vi "rainbow.vi"() -> ()   [LabVIEW 2020]
uses:
  <vilib>/Rock Robotics/SystemInterfaces/DIO/FPGA_DIOPWMChannel.ctl
  Users/Adam/Downloads/bling-main/bling-main/BlingLibrary/ArduinoSerialBling.lvlib
panel:
  out "LED Strip":u32[](array[colorbox])
  out "String Length":u16=144
  in  "milliseconds to wait":u32
  in  "PWM Channel":T1=enum."PWM 9"
  in  "stop":bool
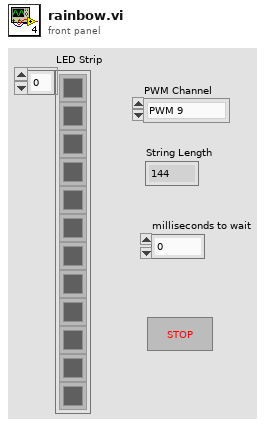
[diagram p1: front panel]
types:
  T1 = typedef "FPGA_DIOPWMChannel.ctl" = enum8{"PWM 0", "PWM 1", "PWM 2", "PWM 3", "PWM 4", "PWM 5", "PWM 6", "PWM 7", "PWM 8", "PWM 9", "PWM MXP 0", "PWM MXP 1", "PWM MXP 2", "PWM MXP 3", "PWM MXP 4", "PWM MXP 5", "PWM MXP 6", "PWM MXP 7", "PWM MXP 8", "PWM MXP 9", "Invalid"}
  T2 = typedef "WPI_PWMDeviceRef.ctl" = cluster{"DeviceStatus":errorcluster, "PWM Channel":T1}
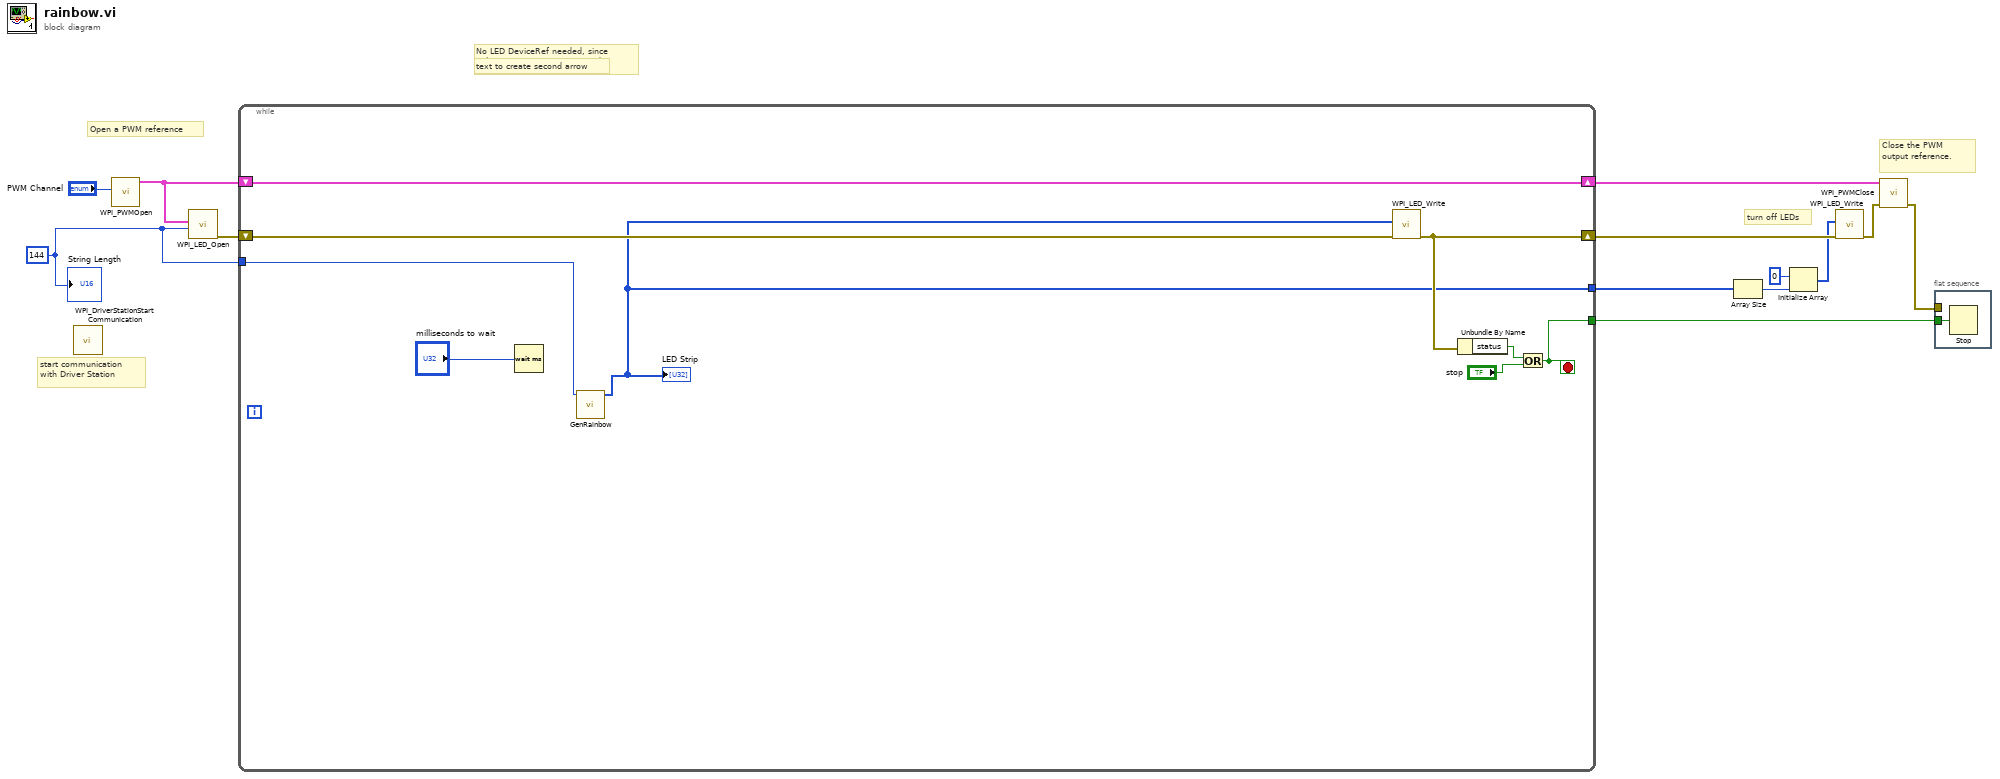
[diagram p0: block diagram]
diagram:
  w1 = u16 144 ("String Length")
  # "turn off LEDs"
  # "No LED DeviceRef needed, since only one LED strip is supported"
  # "Open a PWM reference"
  # "start communication with Driver Station"
  # "Close the PWM output reference."
  # "text to create second arrow"
  n1 = call <vilib>:"WPI_DriverStationStart Communication.vi"() -> ()  [unwired: 3 in, 9 out]
  n2 = call <vilib>:"WPI_PWMOpen.vi"("PWM Channel"="PWM Channel") -> ("PWMDeviceRef"=w10:T2)  [unwired: 9 in, 1 out]
  n3 = call <vilib>:"WPI_LED_Open.vi"("String Length"=w1, "PWMDeviceRef"=w10) -> ("error out"=w11:errorcluster)  [unwired: 9 in]
  n4 = while {
    shift-right: [w19] -> w12
    shift-left: w10 -> [w19]
    tunnel: [w22] -> w13
    shift-right: [w17] -> w8
    shift-left: w11 -> [w18]
    tunnel: w1 -> [w16]
    tunnel: [w14] -> w5
    stop <- w22 stop-if-true
    n5 = Wait (ms)(milliseconds to wait="milliseconds to wait") -> ()  [unwired: 1 out]
    n6 = call "GenRainbow.vi"("NumLeds"=w16) -> ("Rainbow"=w14:u32[])  [unwired: 10 in]
    "LED Strip" <- w14
    n7 = call <vilib>:"WPI_LED_Write.vi"("error in"=w18, "Color Array"=w14) -> ("error out"=w17:errorcluster)  [unwired: 9 in]
    n8 = Unbundle By Name(w17) -> ("status"=w20:bool)
    n9 = Or(x=w20, y="stop") -> (x .or. y?=w22:bool)
  }
  n10 = Array Size(array=w5) -> (size(s)=w6:i32)
  n11 = Initialize Array(u32 0, w6) -> (w3:u32[])
  n12 = call <vilib>:"WPI_LED_Write.vi"("error in"=w8, "Color Array"=w3) -> ("error out"=w7:errorcluster)  [unwired: 9 in]
  n13 = call <vilib>:"WPI_PWMClose.vi"("error in (no error)"=w7, "PWMDeviceRef"=w12) -> ("error out"=w2:errorcluster)  [unwired: 9 in]
  n14 = flat-sequence {
    tunnel: w13 -> [w23]
    tunnel: w2 -> [_]
    frame #0 {
      n15 = Stop(stop? (T)=w23) -> ()
    }
  }
  "String Length" <- w1
